vi "Set_Graph_Properties.vi"(11 "Graph":refnum<vi>) -> ()   [LabVIEW 2020]
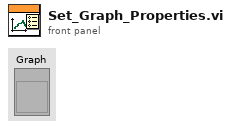
[diagram p1: front panel]
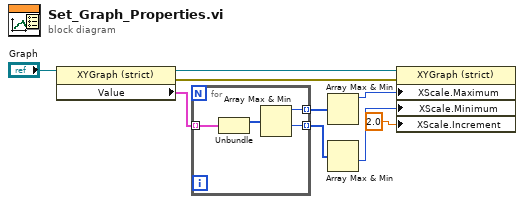
[diagram p0: block diagram]
diagram:
  n1 = property class="XYGraph (strict)"(reference="Graph") -> (reference out=w1:refnum<vi>, error out=w2:errorcluster, "Value"=w3:cluster{i32[], "all rows":dbl[]}[])  [unwired: 1 in]
  n2 = for {
    tunnel: w3 -> [w13] mode=indexing
    tunnel: [w11] -> w9 mode=indexing
    tunnel: [w10] -> w8 mode=indexing
    n3 = Unbundle(w13) -> (w12:i32[])  [unwired: 1 out]
    n4 = Array Max & Min(array=w12) -> (max value=w11:i32, min value=w10:i32)  [unwired: 2 out]
  }
  n5 = Array Max & Min(array=w9) -> (max value=w7:i32)  [unwired: 3 out]
  n6 = Array Max & Min(array=w8) -> (min value=w5:i32)  [unwired: 3 out]
  n7 = property class="XYGraph (strict)"(reference=w1, error in=w2, "XScale.Maximum"=w7, "XScale.Minimum"=w5, "XScale.Increment"=2.0 ("X Scale.Range:Increment")) -> ()  [unwired: 2 out]
